vi "Get_Data.vi"(0 "Divide in":refnum<class "Divide.lvclass">, 11 "Error In":errorcluster) -> (4 "Divide out":refnum<class "Divide.lvclass">, 15 "Error Out":errorcluster)   [LabVIEW 2020, in "Divide.lvclass"]
doc: "Method to get the object data from the UI method."
uses:
  Divide.lvclass
  Arithmetic_Operations/Arithmetic_Operations.lvclass
  Divide.lvclass/Divide.ctl
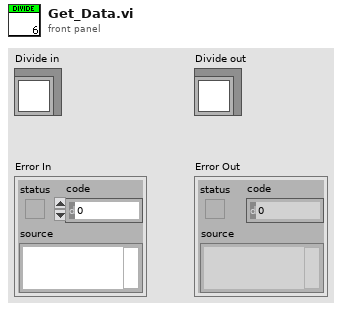
[diagram p1: front panel]
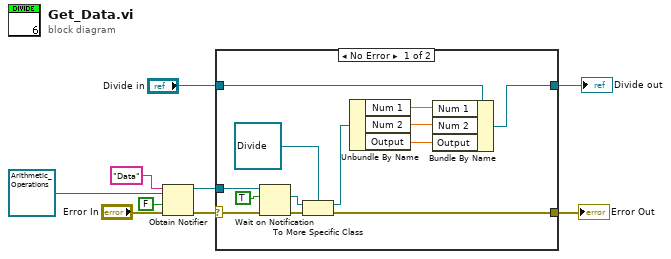
[diagram p0: block diagram]
diagram:
  n1 = Obtain Notifier(name (unnamed)="Data", notification data type=refnum<class "Arithmetic_Operations.lvclass"> refnum ("Arithmetic_Operations.lvclass"), create if not found? (T)=FALSE, error in (no error)="Error In") -> (notifier out=w7:refnum<notifier>, error out=w5:errorcluster)  [unwired: 1 out]
  n2 = case shown="No Error" w5 {
    selector: w5 -> [w17 w24]
    tunnel: [w14 w24] -> w9
    tunnel: [w21 w23] -> w2
    tunnel: "Divide in" -> [w22 w23]
    tunnel: w7 -> [w15 _]
    frame No Error {
      n3 = Wait on Notification(notifier=w15, ignore previous (F)=TRUE, error in (no error)=w17) -> (notification=w13:refnum<class "Arithmetic_Operations.lvclass">, error out=w16:errorcluster)  [unwired: 1 in, 2 out]
      n4 = To More Specific Class(target class=refnum<class "Divide.lvclass"> refnum ("Divide.lvclass"), reference=w13, error in=w16) -> (specific class reference=w12:refnum<class "Divide.lvclass">, error out=w14:errorcluster)
      n5 = Unbundle By Name(w12) -> ("Num 1"=w20:dbl, "Num 2"=w19:dbl, "Output"=w18:dbl)
      n6 = Bundle By Name(cluster=w22, "Num 1"=w20, "Num 2"=w19, "Output"=w18) -> (w21:refnum<class "Divide.lvclass">)
    }
    frame Error {
    }
  }
  "Divide out" <- w2
  "Error Out" <- w9
